vi "List Devices.vi"(8 "error in (no error)":errorcluster, 10 "Filter (Device Description)":string) -> (0 "error out":errorcluster, 2 "Devices":T1[](array[typedef]))   [LabVIEW 2019, in "D2XX-lv.lvlib"]
doc: "List all connected devices that match the Device Description search filter."
uses:
  D2XX-lv.lvlib
  typedefs/Device Info.ctl
  <instrlib>/_D2XX/D2XX/FT_Open_Device_By_Serial_Number.vi
  private/FT_Status to Error.vi
  Open Device (serial number).vi
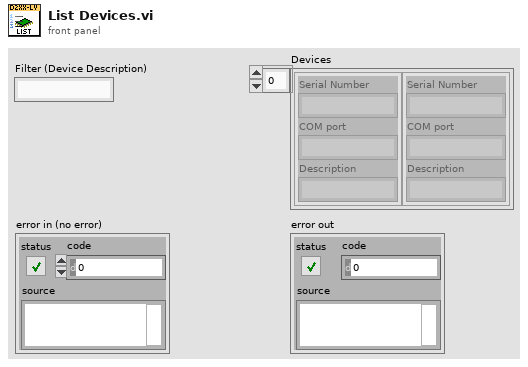
[diagram p1: front panel]
types:
  T1 = typedef "D2XX-lv.lvlib/Device Info.ctl" = cluster{"Serial Number":string, "COM port":string, "Description":string}
  T2 = cluster{"Type":u32, "VID":string, "PID":string, "Serial Number":string, "Description":string}
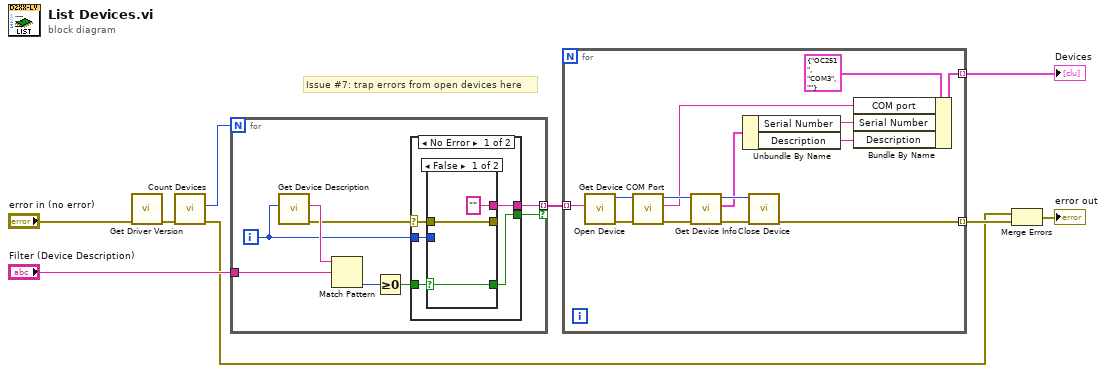
[diagram p0: block diagram]
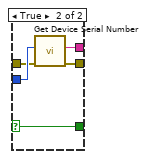
[diagram p2: hidden frame]
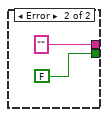
[diagram p3: hidden frame]
diagram:
  # "Issue #7: trap errors from open devices here"
  n1 = call "Get Driver Version.vi"("error in (no error)"="error in (no error)") -> ("error out"=w5:errorcluster)  [unwired: 9 in, 1 out]
  n2 = call "Count Devices.vi"("error in (no error)"=w5) -> ("error out"=w2:errorcluster, "Number of Devices"=w1:i32)  [unwired: 9 in]
  n3 = for {
    N: w1 -> [_]
    tunnel: [w17] -> w4 mode=indexing if=w10
    tunnel: "Filter (Device Description)" -> [w15]
    i -> [w13]
    n4 = call "Get Device Description.vi"("Device Index"=w13) -> ("error out"=w12:errorcluster, "Device Description"=w14:string)  [unwired: 9 in]
    n5 = Match Pattern(string=w14, regular expression=w15) -> (offset past match=w16:i32)  [unwired: 1 in, 3 out]
    n6 = Greater Or Equal To 0?(x=w16) -> (x >= 0?=w11:bool)
    n7 = case shown="No Error" w12 {
      selector: w12 -> [w20 _]
      tunnel: [w22 "" ("Device Serial Number")] -> w17
      tunnel: w13 -> [w21 _]
      tunnel: w11 -> [w19 _]
      tunnel: [w18 FALSE] -> w10
      frame No Error {
        n8 = case shown="False" w19 {
          selector: w19 -> [w25 w27]
          tunnel: ["" ("Device Serial Number") w30] -> w22
          tunnel: w21 -> [_ w29]
          tunnel: w20 -> [w23 w28]
          tunnel: [w25 w27] -> w18
          tunnel: [w23 w26] -> _
          frame False {
          }
          frame True {
            n9 = call "Get Device Serial Number.vi"("error in (no error)"=w28, "Device Index"=w29) -> ("error out"=w26:errorcluster, "Device Serial Number"=w30:string)  [unwired: 8 in]
          }
        }
      }
      frame Error {
      }
    }
  }
  n10 = for {
    tunnel: w4 -> [w44] mode=indexing
    tunnel: [w37] -> w8 mode=indexing
    tunnel: [w43] -> w3 mode=indexing
    n11 = call-poly "Open Device.vi"("Device Serial Number"=w44) -> ("error out"=w45:errorcluster, "Handle"=w46:u64)  [unwired: 9 in]
    n12 = call "Get Device COM Port.vi"("error in (no error)"=w45, "Handle"=w46) -> ("error out"=w41:errorcluster, "COM Port"=w34:string, "Handle out"=w42:u64)  [unwired: 7 in]
    n13 = call "Get Device Info.vi"("error in (no error)"=w41, "Handle"=w42) -> ("error out"=w39:errorcluster, "Device Information"=w33:T2, "Handle out"=w40:u64)  [unwired: 7 in]
    n14 = Unbundle By Name(w33) -> ("Serial Number"=w36:string, "Description"=w35:string)
    n15 = call "Close Device.vi"("error in (no error)"=w39, "Handle"=w40) -> ("error out"=w43:errorcluster)  [unwired: 9 in]
    n16 = Bundle By Name(cluster=T1 {"Serial Number"="OC251", "COM port"="COM3", "Description"=""}, "COM port"=w34, "Serial Number"=w36, "Description"=w35) -> (w37:T1)
  }
  "Devices" <- w8
  n17 = Merge Errors(w2, w3) -> (→"error out":errorcluster)
